vi "(SubVI) Wang 97 Tether Calibration-Calculate Xbd and Xst.vi"(5 "Calibration":T1, 6 "QPD Array (V)":dbl[](array[numeric]), 7 "Stage Position Array (um)":dbl[](array[numeric])) -> (0 "Xbdi Array (nm)":dbl[](array[numeric]), 1 "zbd Array (nm)":dbl[](array[numeric]), 2 "Xbd Array (nm)":dbl[](array[numeric]), 3 "Xst Array (nm)":dbl[](array[numeric]))   [LabVIEW 2014]
uses:
  Calibration.ctl
panel:
  out "Waveform Graph":dbl[][](graph)
  out "Xst (nm)":dbl
  out "Xbd (nm)":dbl
  out "Zbd":dbl
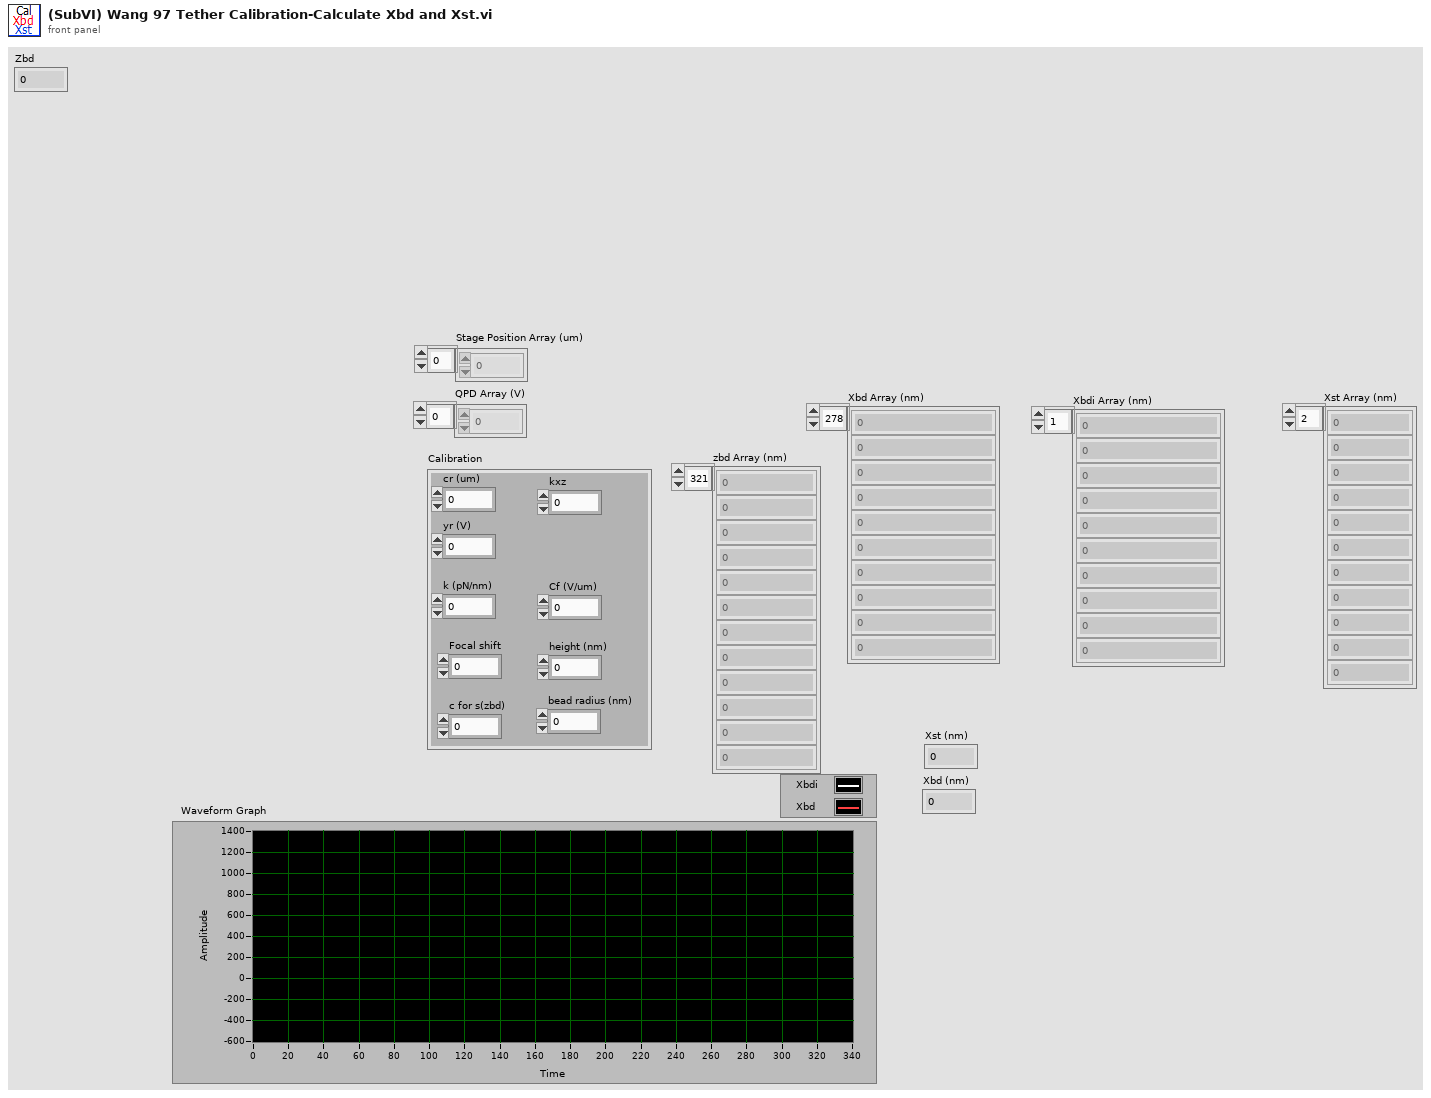
[diagram p1: front panel]
types:
  T1 = typedef "Calibration.ctl" = cluster{"cr (um)":dbl, "yr (V)":dbl, "height (nm)":dbl, "Cf (V/um)":dbl, "kxz":dbl, "k (pN/nm)":dbl, "Focal shift":dbl, "c for s(zbd)":dbl, "bead radius (nm)":dbl}
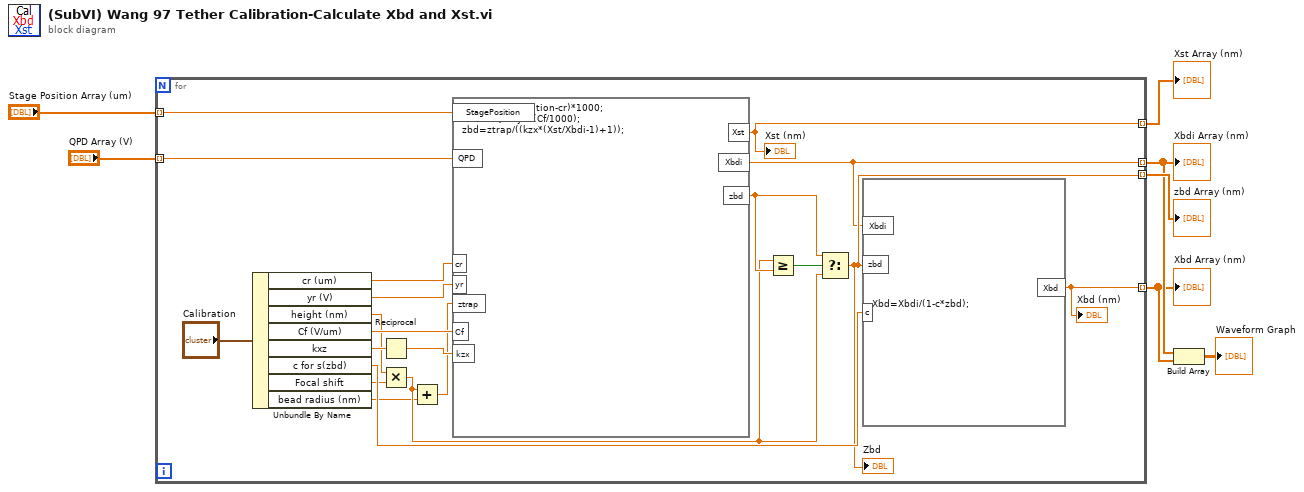
[diagram p0: block diagram]
diagram:
  n1 = for {
    tunnel: "QPD Array (V)" -> [w18] mode=indexing
    tunnel: "Stage Position Array (um)" -> [w17] mode=indexing
    tunnel: [w16] -> w2 mode=indexing
    tunnel: [w15] -> w5 mode=indexing
    tunnel: [w14] -> w4 mode=indexing
    tunnel: [w11] -> w3 mode=indexing
    n2 = Unbundle By Name("Calibration") -> ("cr (um)"=w23:dbl, "yr (V)"=w22:dbl, "height (nm)"=w13:dbl, "Cf (V/um)"=w21:dbl, "kxz"=w20:dbl, "c for s(zbd)"=w19:dbl, "Focal shift"=w12:dbl, "bead radius (nm)"=w9:dbl)
    n3 = Reciprocal(x=w20) -> (1/x=w25:dbl)
    n4 = Multiply(x=w13, y=w12) -> (x*y=w10:dbl)
    n5 = Add(x=w10, y=w9) -> (x+y=w8:dbl)
    n6 = formula code="Xst=(StagePosition-cr)*1000;\nXbdi=(QPD-yr)/(Cf/1000);\nzbd=ztrap/((kzx*(Xst/Xbdi-1)+1));"("ztrap"=w8, "kzx"=w25, "StagePosition"=w17, "cr"=w23, "Cf"=w21, "QPD"=w18, "yr"=w22) -> ("zbd"=w27:dbl, "Xbdi"=w11:dbl, "Xst"=w15:dbl)
    "Xst (nm)" <- w15
    n7 = Greater Or Equal?(x=w10, y=w27) -> (x >= y?=w26:bool)
    n8 = Select(t=w27, s=w26, f=w10) -> (s? t:f=w14:dbl)
    "Zbd" <- w14
    n9 = formula code="Xbd=Xbdi/(1-c*zbd);"("Xbdi"=w11, "zbd"=w14, "c"=w19) -> ("Xbd"=w16:dbl)
    "Xbd (nm)" <- w16
  }
  "Xbd Array (nm)" <- w2
  "Xst Array (nm)" <- w5
  "zbd Array (nm)" <- w4
  "Xbdi Array (nm)" <- w3
  n10 = Build Array(w3, w2) -> (→"Waveform Graph":dbl[][])
